vi "R=Left_Arm.vi"(9 "Matrix":T1 format="%.3f", 11 "Command":string="Reference") -> (0 "error out":errorcluster, 2 "Joints":dbl[](array[numeric])=[0.0, -45.0, 0.0, 45.0, 0.0, 90.0, 0.0], 3 "Matrix":T1 format="%.3f")   [LabVIEW 2013]
uses:
  <vilib>/Analysis/Matrix/Datatypes/RealMatrix.ctl
  ROS/Code/SubVIs/BaxterSide.ctl
  ROS/Code/Console/Servers/ServerSubs/(nist) Arm Globals.vi
  <vilib>/Analysis/Matrix/Numeric/Multiply/Multiply - RM,RM.vi
  <vilib>/Analysis/baseanly.llb/Real Inverse Matrix.vi
  <vilib>/Analysis/Matrix/NI_Matrix.lvlib
  <vilib>/Analysis/NI_AALBase.lvlib
panel:
  out "Left tool":T1 format="%.3f"
  in  "Ref Point":dbl[](array[numeric])=[45.0, -45.0, 0.0, 90.0, 0.0, 45.0, 0.0]
  in  "Offset out":T2
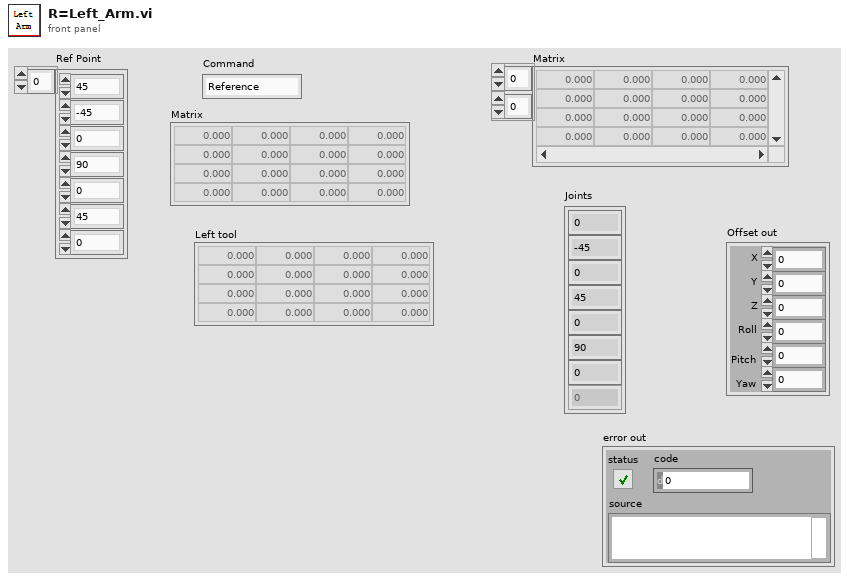
[diagram p1: front panel]
types:
  T1 = typedef "NI_Matrix.lvlib/RealMatrix.ctl" = dbl[][]
  T2 = cluster{"X":dbl, "Y":dbl, "Z":dbl, "Roll":dbl, "Pitch":dbl, "Yaw":dbl}
  T3 = typedef "BaxterSide.ctl" = enum16{"left", "right"}
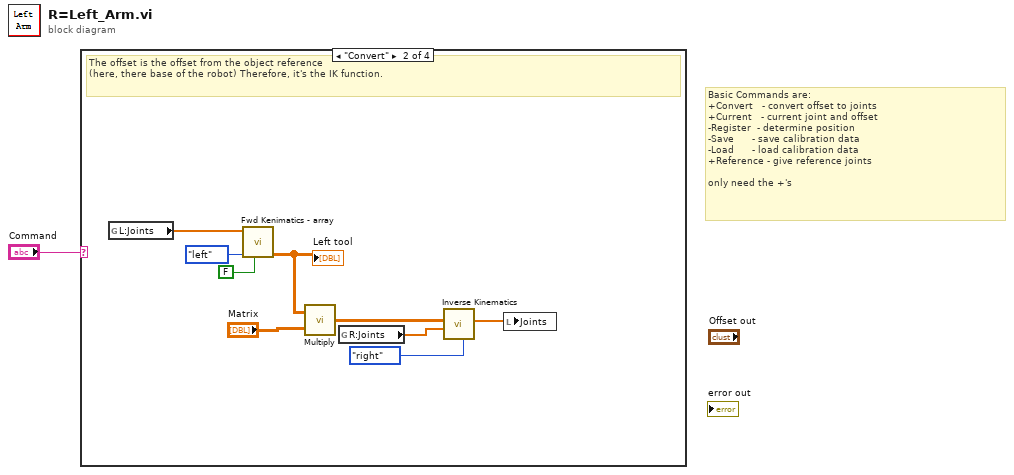
[diagram p0: block diagram]
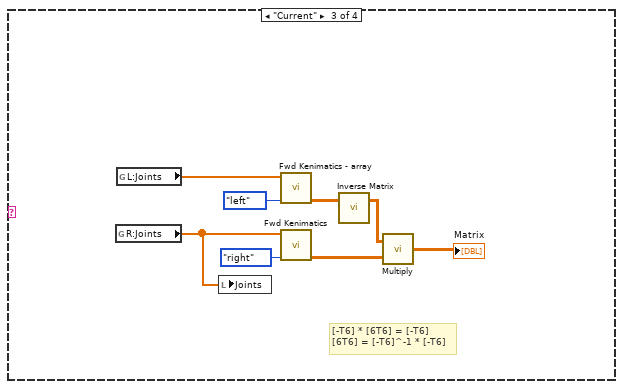
[diagram p3: hidden frame]
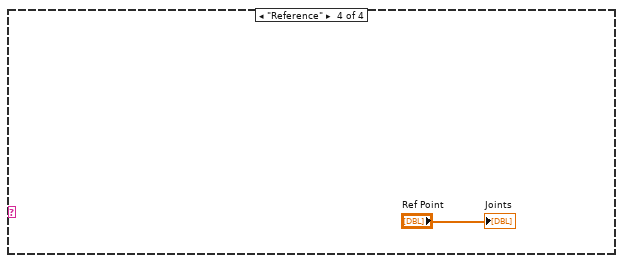
[diagram p4: hidden frame]
diagram:
  # "Basic Commands are:\n+Convert   - convert offset to joints\n+Current   - current joint and offset\n-Register  - determine position\n-Save      - save calibration data\n-Load      - load calibration data\n+Reference - give reference joints\n\nonly need the +'s"
  n1 = case shown="\"Convert\"" "Command" {
    frame Default {
    }
    frame "Convert" {
      # "The offset is the offset from the object reference\n(here, there base of the robot) Therefore, it's the IK function."
      n2 = global read "(nist) Arm Globals.vi" "L:Joints"() -> (w4:dbl[])
      n3 = call "Fwd Kenimatics - array.vi"("Make Vertical"=FALSE, "Side"=BaxterSide."left", "Joints"=w4) -> ("Matrix"=w7:T1)  [unwired: 7 in, 1 out]
      "Left tool" <- w7
      n4 = call-poly <vilib>:"Multiply.vi"("Real Matrix B"="Matrix", "Real Matrix A"=w7) -> ("A * B"=w6:T1)
      n5 = global read "(nist) Arm Globals.vi" "R:Joints"() -> (w5:dbl[])
      n6 = call "Inverse Kinematics.vi"("Side"=BaxterSide."right", "Start"=w5, "Goal-matrix"=w6) -> ("J"=w9:dbl[])  [unwired: 5 in, 3 out]
      n7 = local write "Joints"(w9) -> ()
    }
    frame "Current" {
      # "[-T6] * [6T6] = [-T6]\n[6T6] = [-T6]^-1 * [-T6]"
      n8 = global read "(nist) Arm Globals.vi" "R:Joints"() -> (w11:dbl[])
      n9 = global read "(nist) Arm Globals.vi" "L:Joints"() -> (w12:dbl[])
      n10 = local write "Joints"(w11) -> ()
      n11 = call "Fwd Kenimatics - array.vi"("Side"=BaxterSide."left", "Joints"=w12) -> ("Matrix"=w16:T1)  [unwired: 8 in, 1 out]
      n12 = call-poly "Fwd Kenimatics.vi"("Side"=BaxterSide."right", "Joints"=w11) -> ("Matrix"=w15:T1)  [unwired: 8 in, 1 out]
      n13 = call-poly <vilib>:"Inverse Matrix.vi"("Input Matrix"=w16) -> ("Inverse Matrix"=w13:T1)  [unwired: 1 in, 1 out]
      n14 = call-poly <vilib>:"Multiply.vi"("Real Matrix B"=w15, "Real Matrix A"=w13) -> ("A * B"=→"Matrix":T1)
    }
    frame "Reference" {
      "Joints" <- "Ref Point"
    }
  }
